vi "Logging Message Loop.vi"(8 "error in (no error)":errorcluster, 10 "Data Queue":refnum<queue>, 11 "Message Queues":T1) -> (0 "error out":errorcluster)   [LabVIEW 2016, in "Logging.lvlib"]
doc: "The message loop subVI to handle messages pertaining to logging data."
uses:
  Logging.lvlib
  support/Message Queue/All Message Queues.ctl
  support/Message Queue/Message Cluster.ctl
  Logging Configuration.ctl
  Logging State.ctl
  support/Message Queue/Enqueue Message (Single).vi
  <vilib>/Utility/error.llb/Error Cluster From Error Code.vi
  <vilib>/ErrorRing/Error Ring.xnode
  support/Message Queue/Message Queue.lvlib
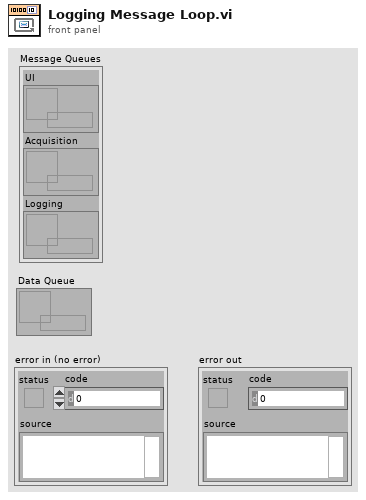
[diagram p1: front panel]
types:
  T1 = typedef "Message Queue.lvlib/All Message Queues.ctl" = cluster{"UI":refnum<queue>, "Acquisition":refnum<queue>, "Logging":refnum<queue>}
  T2 = typedef "Logging.lvlib/Logging State.ctl" = cluster{"State":enum16{"Logging", "Not Logging", "Idle"}, "Samples to Save":u32, "Force Trigger":bool}
  T3 = typedef "Logging.lvlib/Logging Configuration.ctl" = cluster{"Log File Base Path":path, "TDMS File Reference":refnum<k34>, "Samples to Save":u32, "Trigger - Time":u32, "Trigger - Threshold":dbl, "Trigger - Channel":u32, "Enable Time Trigger":bool, "Enable Threshold Trigger":bool, "Always Log":bool}
  T4 = enum16{"open", "open or create", "create or replace", "create", "open (read-only)"}
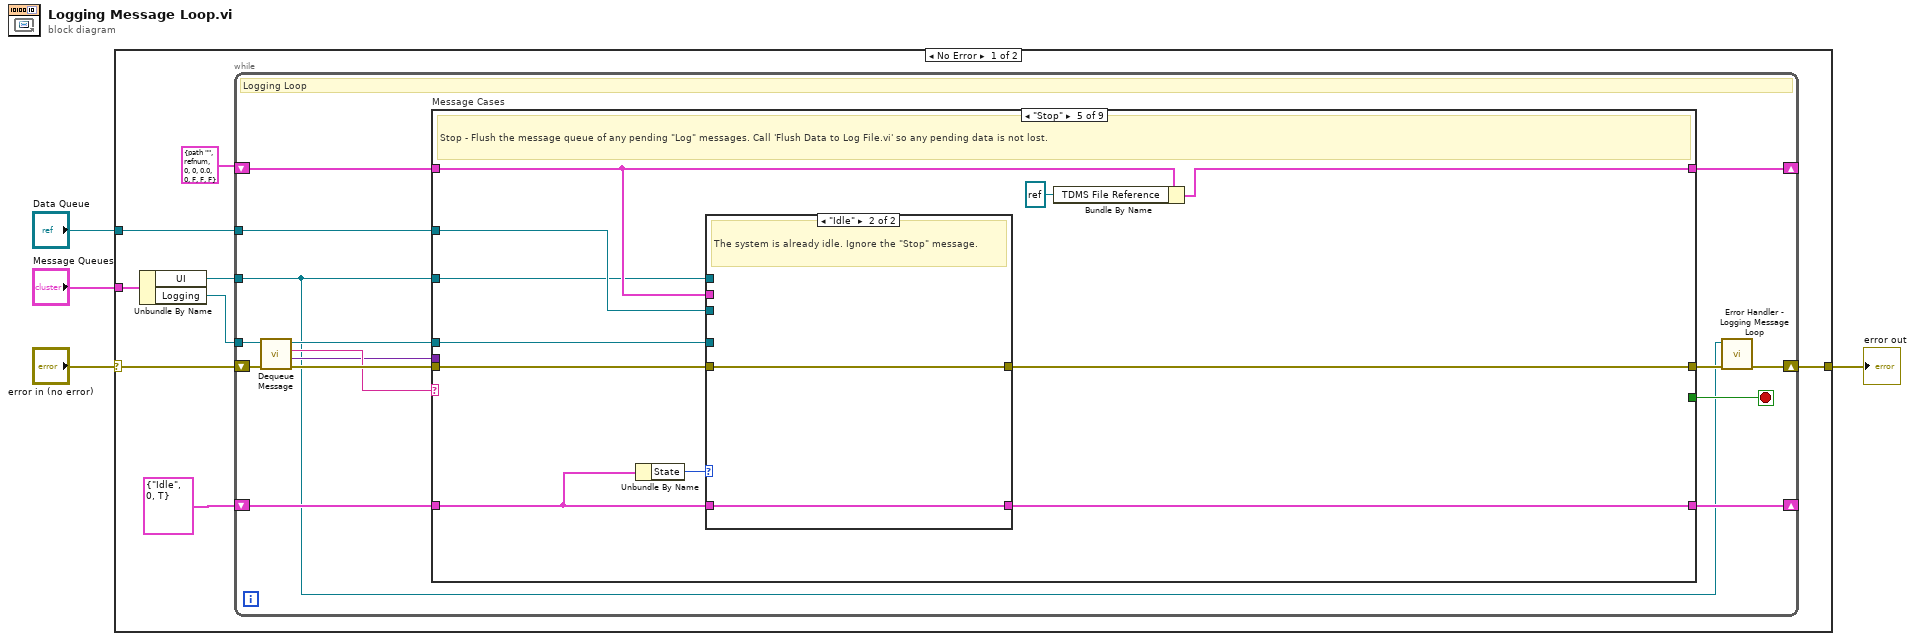
[diagram p0: block diagram]
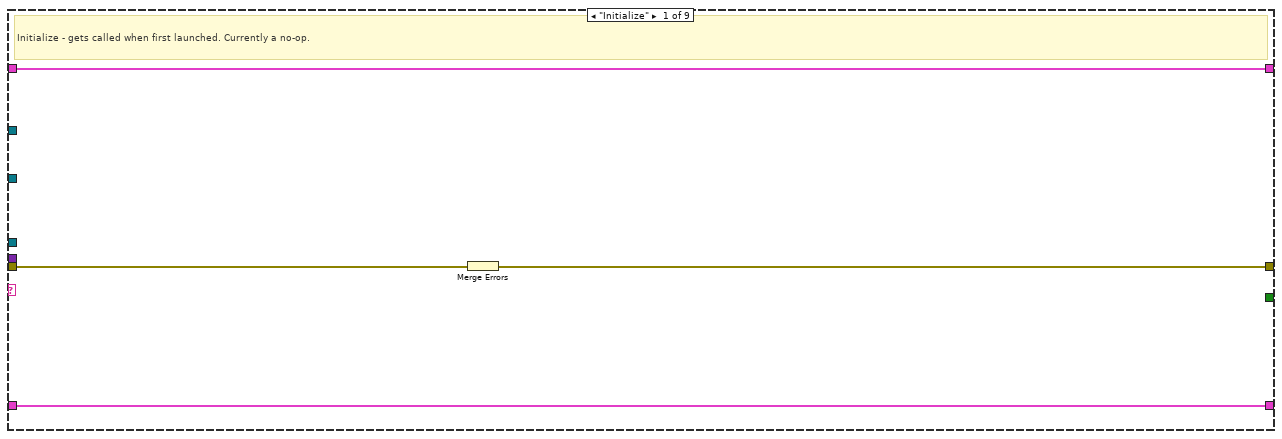
[diagram p2: hidden frame]
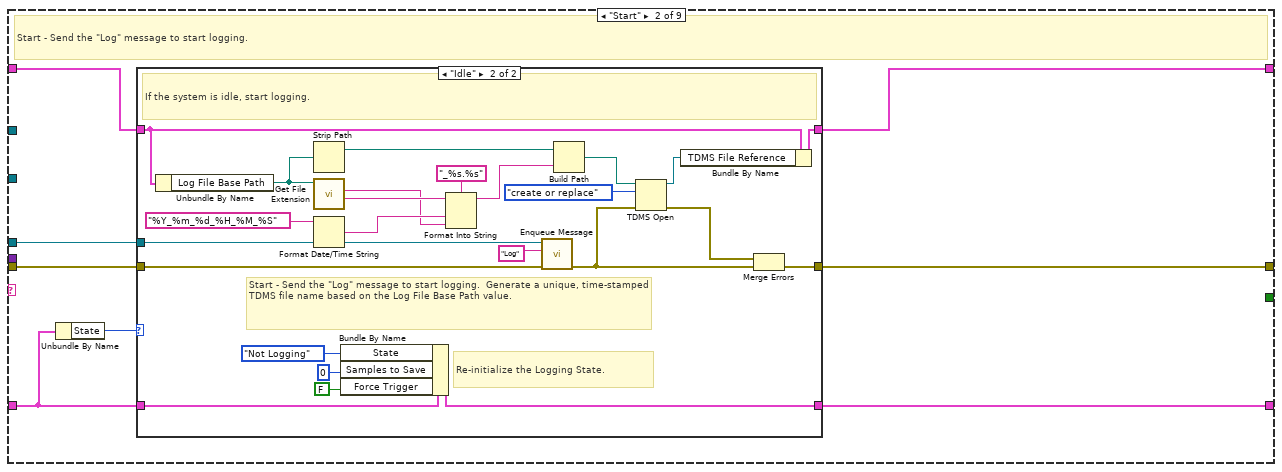
[diagram p3: hidden frame]
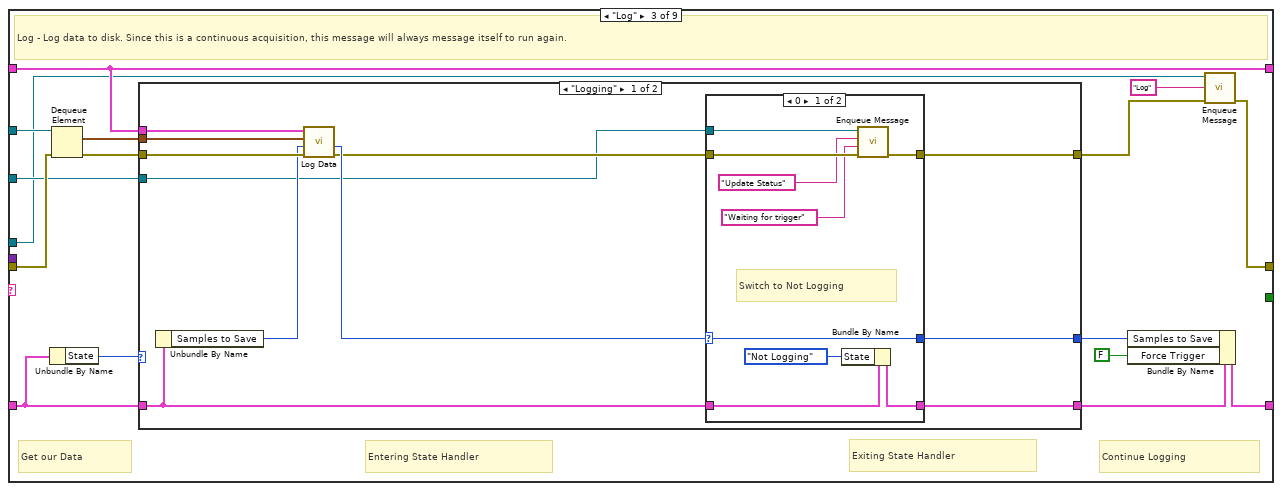
[diagram p5: hidden frame]
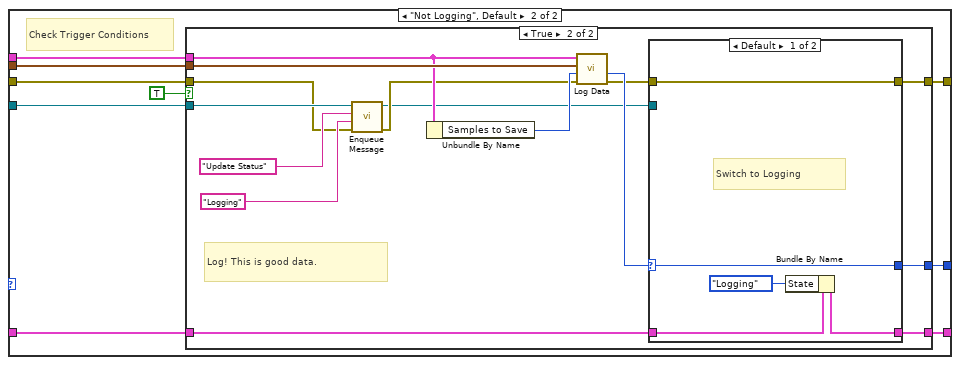
[diagram p7: hidden frame]
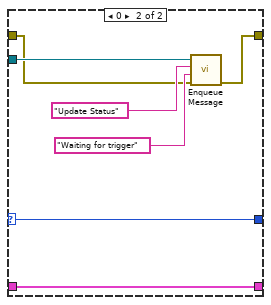
[diagram p9: hidden frame]
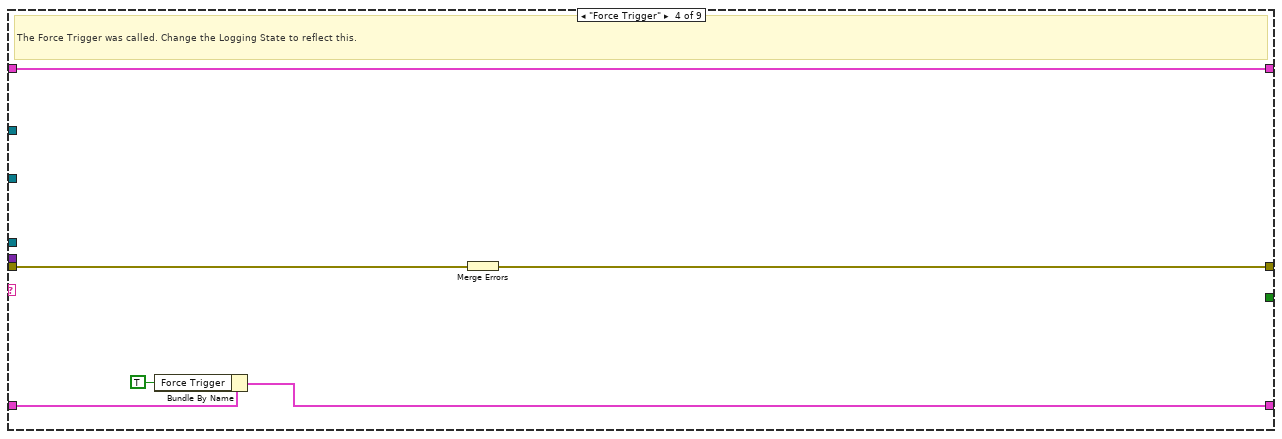
[diagram p10: hidden frame]
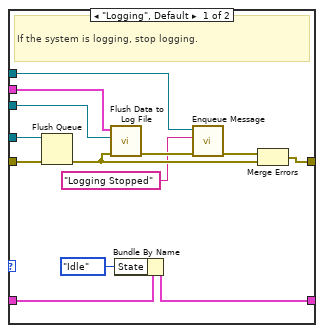
[diagram p11: hidden frame]
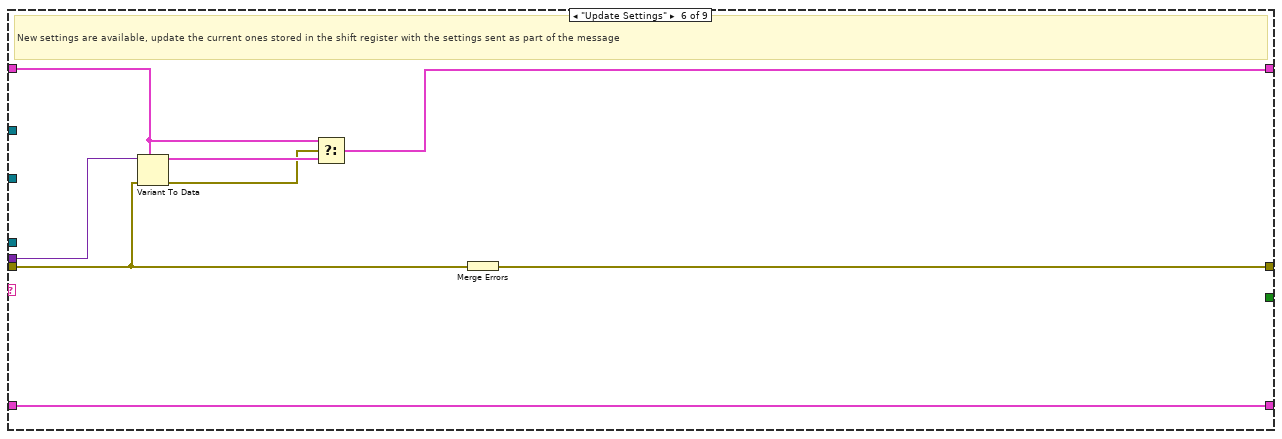
[diagram p12: hidden frame]
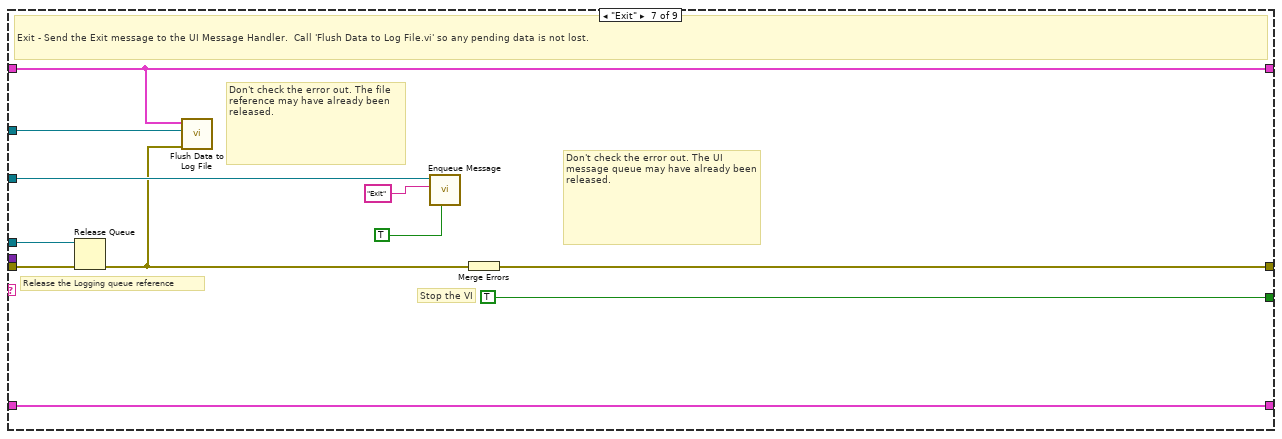
[diagram p13: hidden frame]
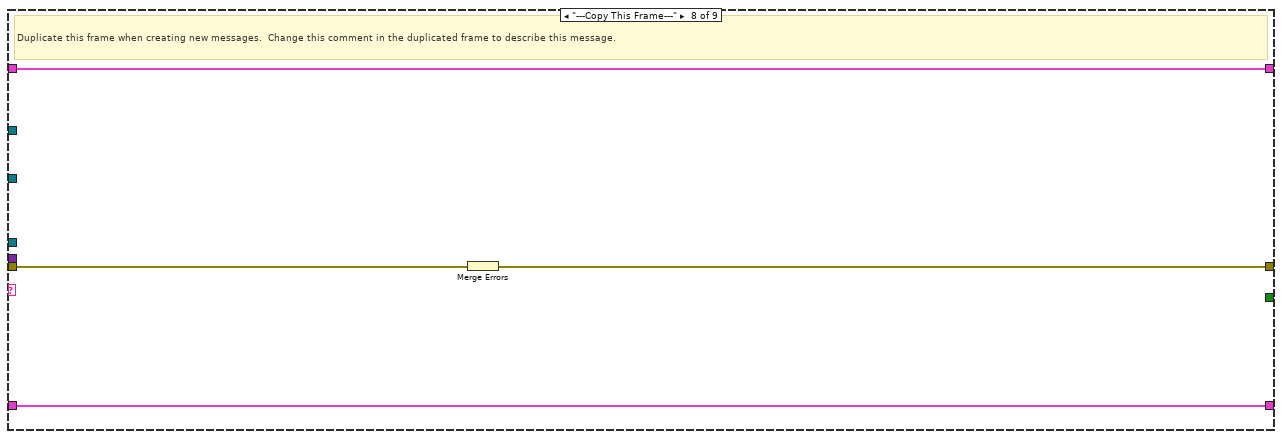
[diagram p14: hidden frame]
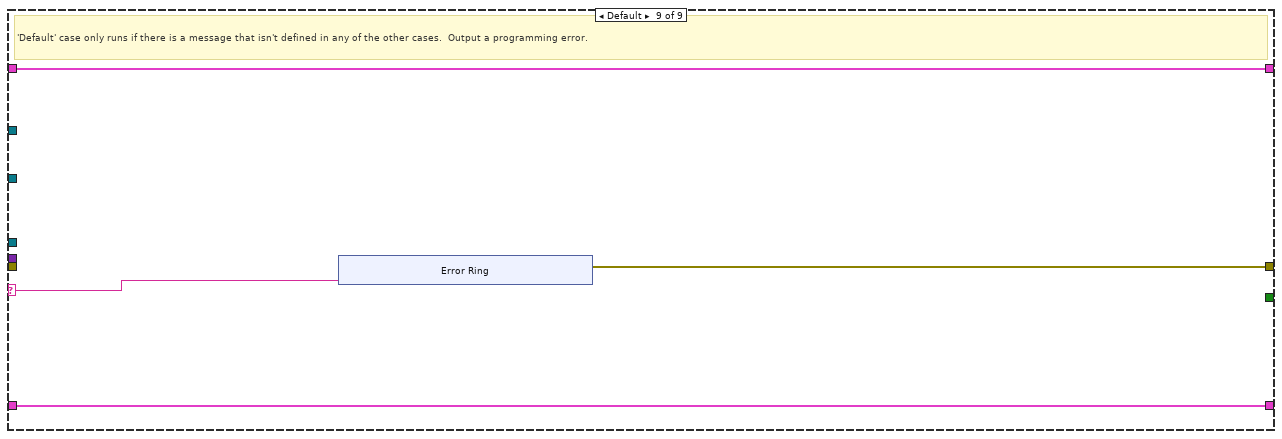
[diagram p15: hidden frame]
diagram:
  n1 = case shown="No Error" "error in (no error)" {
    selector: "error in (no error)" -> [w8 w210]
    tunnel: "Message Queues" -> [w12 _]
    tunnel: [w10 w210] -> w3
    tunnel: "Data Queue" -> [w7 _]
    frame No Error {
      n2 = Unbundle By Name(w12) -> ("UI"=w6:refnum<queue>, "Logging"=w11:refnum<queue>)
      n3 = while {
        tunnel: w11 -> [w19]
        shift-right: [w26] -> _
        shift-left: T3 {"Log File Base Path"=path "", "TDMS File Reference"=refnum, "Samples to Save"=0, "Trigger - Time"=0, "Trigger - Threshold"=0.0, "Trigger - Channel"=0, "Enable Time Trigger"=FALSE, "Enable Threshold Trigger"=FALSE, "Always Log"=FALSE} ("Logging Configuration") -> [w27]
        shift-right: [w14] -> w10
        shift-left: w8 -> [w24]
        tunnel: w6 -> [w13]
        tunnel: w7 -> [w18]
        shift-right: [w16] -> _
        shift-left: T2 {"State"=enum."Idle", "Samples to Save"=0, "Force Trigger"=TRUE} -> [w17]
        stop <- w25 stop-if-true
        # "Logging Loop"
        n4 = call "Dequeue Message.vi"("error in (no error)"=w24, "Message Queue"=w19) -> ("error out"=w23:errorcluster, "Message Data"=w21:variant, "Message"=w22:string, "dup Message Queue"=w20:refnum<queue>)  [unwired: 6 in]
        n5 = case "Message Cases" shown="\"Stop\"" w22 {
          selector: w22 -> [_ _ _ _ _ _ _ _ w199]
          tunnel: w20 -> [_ w38 w70 _ w158 _ w188 _ _]
          tunnel: w23 -> [w29 w37 w80 w149 w159 w177 w191 w198 _]
          tunnel: [w31 w39 w82 w147 w160 w183 w193 w196 w200] -> w15
          tunnel: w27 -> [w30 w36 w75 w148 w155 w181 w187 w197 w202]
          tunnel: [w30 w35 w75 w148 w157 w178 w187 w197 w202] -> w26
          tunnel: [_ _ _ _ _ _ TRUE _ _] -> w25
          tunnel: w21 -> [_ _ _ _ _ w182 _ _ _]
          tunnel: w13 -> [_ _ w74 _ w153 _ w192 _ _]
          tunnel: w18 -> [_ _ w71 _ w154 _ w186 _ _]
          tunnel: w17 -> [w28 w33 w78 w146 w151 w176 w184 w195 w201]
          tunnel: [w28 w34 w73 w145 w150 w176 w184 w195 w201] -> w16
          frame "Initialize" {
            # "Initialize - gets called when first launched. Currently a no-op."
            n6 = Merge Errors(w29) -> (w31:errorcluster)
          }
          frame "Start" {
            # "Start - Send the \"Log\" message to start logging."
            n7 = Unbundle By Name(w33) -> ("State"=w32:enum16{"Logging", "Not Logging", "Idle"})
            n8 = case shown="\"Idle\"" w32 {
              tunnel: [w41 w66] -> w39
              tunnel: w38 -> [_ w65]
              tunnel: w37 -> [w41 w63]
              tunnel: w36 -> [w42 w54]
              tunnel: [w42 w51] -> w35
              tunnel: w33 -> [w40 w47]
              tunnel: [w40 w46] -> w34
              frame "Logging", Default {
                # "The system is already running. Ignore the \"Start\" message."
              }
              frame "Idle" {
                # "Re-initialize the Logging State."
                # "Start - Send the \"Log\" message to start logging.  Generate a unique, time-stamped TDMS file name based on the Log File Base Path value."
                # "If the system is idle, start logging."
                n9 = Unbundle By Name(w54) -> ("Log File Base Path"=w61:path)
                n10 = Strip Path(path=w61) -> (stripped path=w60:path)  [unwired: 1 out]
                n11 = call <vilib>:"Get File Extension.vi"("file"=w61) -> ("filename without extension"=w59:string, "lowercase file extension"=w56:string)  [unwired: 6 in, 3 out]
                n12 = Format Date/Time String(time format string (%c)="%Y_%m_%d_%H_%M_%S") -> (date/time string=w57:string)  [unwired: 2 in]
                n13 = Bundle By Name(cluster=w47, "State"=enum16{"Logging", "Not Logging"}."Not Logging", "Samples to Save"=u32 0 ("Reads to Save"), "Force Trigger"=FALSE) -> (w46:T2)
                n14 = Format Into String(format string="_%s.%s", initial string=w59, w57, w56) -> (resulting string=w55:string)  [unwired: 1 in, 1 out]
                n15 = call-poly "Enqueue Message.vi"("error in (no error)"=w63, "Message"="Log", "Message Queue"=w65) -> ("error out"=w49:errorcluster)  [unwired: 7 in, 1 out]
                n16 = Build Path(base path=w60, name or relative path=w55) -> (appended path=w52:path)
                n17 = TDMS Open(8:w49, 10:T4."create or replace" ("operation (0:open)"), 11:w52) -> (0:w48:errorcluster, 3:w53:refnum<k34>)  [unwired: 4 in]
                n18 = Bundle By Name(cluster=w54, "TDMS File Reference"=w53) -> (w51:T3)
                n19 = Merge Errors(w48, w49) -> (w66:errorcluster)
              }
            }
          }
          frame "Log" {
            # "Exiting State Handler"
            # "Continue Logging"
            # "Entering State Handler"
            # "Get our Data"
            # "Log - Log data to disk. Since this is a continuous acquisition, this message will always message itself to run again."
            n20 = Unbundle By Name(w78) -> ("State"=w79:enum16{"Logging", "Not Logging", "Idle"})
            n21 = Dequeue Element(queue=w71, error in (no error)=w80) -> (element=w77:waveform(dbl)[], error out=w76:errorcluster)  [unwired: 1 in, 2 out]
            n22 = case shown="\"Logging\"" w79 {
              tunnel: [w87 w114] -> w69
              tunnel: w78 -> [w88 w112]
              tunnel: w77 -> [w92 w107]
              tunnel: w76 -> [w91 w108]
              tunnel: w75 -> [w93 w106]
              tunnel: w74 -> [w83 w111]
              tunnel: [w84 w113] -> w67
              tunnel: [w86 w110] -> w68
              frame "Logging" {
                n23 = Unbundle By Name(w88) -> ("Samples to Save"=w90:u32)
                n24 = call "Log Data.vi"("error in (no error)"=w91, "Samples to Save In"=w90, "Data"=w92, "Logging Configuration"=w93) -> ("error out"=w85:errorcluster, "Samples to Save Out"=w89:u32)  [unwired: 6 in]
                n25 = case shown="0" w89 {
                  selector: w89 -> [w99 w105]
                  tunnel: w85 -> [w97 w104]
                  tunnel: [w98 w104] -> w84
                  tunnel: w88 -> [w101 w103]
                  tunnel: [w100 w103] -> w87
                  tunnel: [w99 w105] -> w86
                  tunnel: w83 -> [w94 _]
                  frame 0 {
                    # "Switch to Not Logging"
                    n26 = Bundle By Name(cluster=w101, "State"=enum16{"Logging", "Not Logging"}."Not Logging") -> (w100:T2)
                    n27 = call-poly "Enqueue Message.vi"("error in (no error)"=w97, "Message Data"="Waiting for trigger" ("Waiting for trigger"), "Message"="Update Status", "Message Queue"=w94) -> ("error out"=w98:errorcluster)  [unwired: 6 in, 1 out]
                  }
                  frame Default {
                    # "Continue in our same State."
                  }
                }
              }
              frame "Not Logging", Default {
                # "Check Trigger Conditions"
                n28 = case shown="True" TRUE {
                  tunnel: w108 -> [w115 w125]
                  tunnel: w107 -> [_ w131]
                  tunnel: w106 -> [_ w130]
                  tunnel: w112 -> [w116 w121]
                  tunnel: [w116 w120] -> w114
                  tunnel: [w115 w118] -> w113
                  tunnel: w111 -> [_ w129]
                  tunnel: [_ w122] -> w110
                  frame False {
                  }
                  frame True {
                    # "Log! This is good data."
                    n29 = call-poly "Enqueue Message.vi"("error in (no error)"=w125, "Message Data"="Logging" ("Logging"), "Message"="Update Status", "Message Queue"=w129) -> ("error out"=w124:errorcluster, "dup Message Queue"=w117:refnum<queue>)  [unwired: 6 in]
                    n30 = Unbundle By Name(w130) -> ("Samples to Save"=w126:u32)
                    n31 = call "Log Data.vi"("error in (no error)"=w124, "Samples to Save In"=w126, "Data"=w131, "Logging Configuration"=w130) -> ("error out"=w119:errorcluster, "Samples to Save Out"=w123:u32)  [unwired: 6 in]
                    n32 = case shown="Default" w123 {
                      selector: w123 -> [w136 w143]
                      tunnel: [w136 w143] -> w122
                      tunnel: [w133 w142] -> w120
                      tunnel: w121 -> [w134 w142]
                      tunnel: w119 -> [w132 w138]
                      tunnel: [w132 w137] -> w118
                      tunnel: w117 -> [_ w141]
                      frame Default {
                        # "Switch to Logging"
                        n33 = Bundle By Name(cluster=w134, "State"=enum16{"Logging", "Not Logging"}."Logging") -> (w133:T2)
                      }
                      frame 0 {
                        n34 = call-poly "Enqueue Message.vi"("error in (no error)"=w138, "Message Data"="Waiting for trigger" ("Waiting for trigger"), "Message"="Update Status", "Message Queue"=w141) -> ("error out"=w137:errorcluster)  [unwired: 6 in, 1 out]
                      }
                    }
                  }
                }
              }
            }
            n35 = Bundle By Name(cluster=w69, "Samples to Save"=w68, "Force Trigger"=FALSE) -> (w73:T2)
            n36 = call-poly "Enqueue Message.vi"("error in (no error)"=w67, "Message"="Log", "Message Queue"=w70) -> ("error out"=w82:errorcluster)  [unwired: 7 in, 1 out]
          }
          frame "Force Trigger" {
            # "The Force Trigger was called. Change the Logging State to reflect this."
            n37 = Bundle By Name(cluster=w146, "Force Trigger"=TRUE) -> (w145:T2)
            n38 = Merge Errors(w149) -> (w147:errorcluster)
          }
          frame "Stop" {
            # "Stop - Flush the message queue of any pending \"Log\" messages. Call 'Flush Data to Log File.vi' so any pending data is not lost."
            n39 = Unbundle By Name(w151) -> ("State"=w152:enum16{"Logging", "Not Logging", "Idle"})
            n40 = case shown="\"Idle\"" w152 {
              tunnel: [w173 w175] -> w160
              tunnel: w159 -> [w172 w175]
              tunnel: w158 -> [w171 _]
              tunnel: w155 -> [w170 _]
              tunnel: w154 -> [w169 _]
              tunnel: w153 -> [w165 _]
              tunnel: w151 -> [w163 w174]
              tunnel: [w162 w174] -> w150
              frame "Logging", Default {
                # "If the system is logging, stop logging."
                n41 = Flush Queue(queue=w171, error in (no error)=w172) -> (error out=w168:errorcluster)  [unwired: 2 out]
                n42 = call "Flush Data to Log File.vi"("error in (no error)"=w168, "Data Queue"=w169, "Logging Configuration"=w170) -> ("error out"=w167:errorcluster)  [unwired: 8 in]
                n43 = Bundle By Name(cluster=w163, "State"=enum16{"Logging", "Not Logging", "Idle"}."Idle") -> (w162:T2)
                n44 = call-poly "Enqueue Message.vi"("error in (no error)"=w167, "Message"="Logging Stopped", "Message Queue"=w165) -> ("error out"=w166:errorcluster)  [unwired: 7 in, 1 out]
                n45 = Merge Errors(w166, w168) -> (w173:errorcluster)
              }
              frame "Idle" {
                # "The system is already idle. Ignore the \"Stop\" message."
              }
            }
            n46 = Bundle By Name(cluster=w155, "TDMS File Reference"=refnum<k34> refnum ("tdms file out")) -> (w157:T3)
          }
          frame "Update Settings" {
            # "New settings are available, update the current ones stored in the shift register with the settings sent as part of the message"
            n47 = Variant To Data(error in=w177, type=w181, Variant=w182) -> (data=w180:T3, error out=w179:errorcluster)
            n48 = Select(t=w181, s=w179, f=w180) -> (s? t:f=w178:T3)
            n49 = Merge Errors(w177) -> (w183:errorcluster)
          }
          frame "Exit" {
            # "Don't check the error out. The file reference may have already been released."
            # "Release the Logging queue reference"
            # "Don't check the error out. The UI message queue may have already been released."
            # "Stop the VI"
            # "Exit - Send the Exit message to the UI Message Handler.  Call 'Flush Data to Log File.vi' so any pending data is not lost."
            n50 = Release Queue(queue=w188, error in (no error)=w191) -> (error out=w185:errorcluster)  [unwired: 1 in, 2 out]
            n51 = call "Flush Data to Log File.vi"("error in (no error)"=w185, "Data Queue"=w186, "Logging Configuration"=w187) -> ()  [unwired: 8 in, 1 out]
            n52 = call-poly "Enqueue Message.vi"("Priority Message? (F)"=TRUE, "Message"="Exit", "Message Queue"=w192) -> ()  [unwired: 7 in, 2 out]
            n53 = Merge Errors(w185) -> (w193:errorcluster)
          }
          frame "---Copy This Frame---" {
            # "Duplicate this frame when creating new messages.  Change this comment in the duplicated frame to describe this message."
            n54 = Merge Errors(w198) -> (w196:errorcluster)
          }
          frame Default {
            # "'Default' case only runs if there is a message that isn't defined in any of the other cases.  Output a programming error."
            n55 = xnode "Error Ring"("parameter 0"=w199) -> ("error out"=w200:errorcluster)
          }
        }
        n56 = call "Error Handler - Logging Message Loop.vi"("error in (no error)"=w15, "Message Queue"=w13) -> ("dup error in"=w14:errorcluster)  [unwired: 8 in, 1 out]
      }
    }
    frame Error {
    }
  }
  "error out" <- w3
